vi "Sudoku Calculation.vi"(8 "error in (no error)":errorcluster, 11 "Sudoku Class in":refnum<class "Sudoku Class.lvclass">) -> (0 "error out":errorcluster, 3 "Sudoku Class out":refnum<class "Sudoku Class.lvclass">)   [LabVIEW 2015, in "Sudoku Library.lvlib" / "Sudoku Class.lvclass"]
doc: "Created IvanLis by LabVIEW Portal\nProfile: http://labviewportal.org/memberlist.php?mode=viewprofile&u=987\neMail: IvanLisanov@gMail.com\nTelegram: https://t.me/IvanLis"
uses:
  Sudoku Class.lvclass
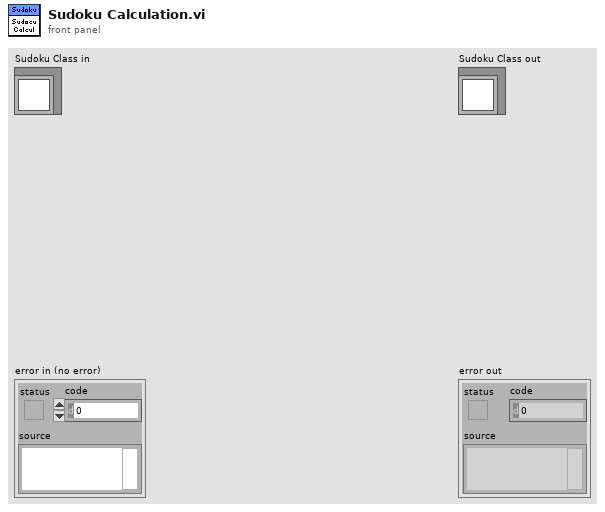
[diagram p1: front panel]
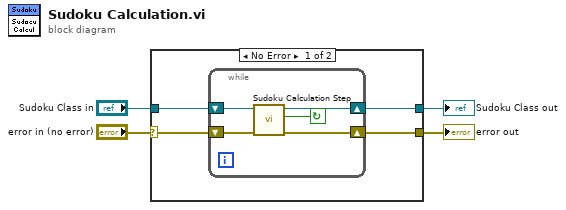
[diagram p0: block diagram]
diagram:
  n1 = case shown="No Error" "error in (no error)" {
    selector: "error in (no error)" -> [w6 w15]
    tunnel: [w5 w15] -> w3
    tunnel: [w7 w14] -> w1
    tunnel: "Sudoku Class in" -> [w8 w14]
    frame No Error {
      n2 = while {
        shift-right: [w12] -> w7
        shift-left: w8 -> [w13]
        shift-right: [w10] -> w5
        shift-left: w6 -> [w11]
        stop <- w9 continue-if-true
        n3 = call "Sudoku Calculation Step.vi"("error in (no error)"=w11, "Sudoku Class in"=w13) -> ("error out"=w10:errorcluster, "Is Modify"=w9:bool, "Sudoku Class out"=w12:refnum<class "Sudoku Class.lvclass">)  [unwired: 7 in]
      }
    }
    frame Error {
    }
  }
  "error out" <- w3
  "Sudoku Class out" <- w1
